vi "vectorAdd.vi"(2 "b":cluster{"xPos":dbl, "yPos":dbl, "Theta":dbl}={"xPos"=nan, "yPos"=nan, "Theta"=nan}, 3 "operation":enum16{"Subtract", "Add"}(ring), 4 "a":cluster{"xPos":dbl, "yPos":dbl, "Theta":dbl}={"xPos"=nan, "yPos"=nan, "Theta"=nan}) -> (1 "a +/- b":cluster{"xPos":dbl, "yPos":dbl, "Theta":dbl}={"xPos"=nan, "yPos"=nan, "Theta"=nan})   [LabVIEW 2016]
uses:
  <vilib>/Analysis/coordinate.llb/Angle Units.ctl
  <vilib>/Analysis/coordinate.llb/Angle Range (Degree).ctl
  <vilib>/Analysis/coordinate.llb/Wrap Angle (scalar).vi
  <vilib>/Analysis/NI_AAL_Angle.lvlib
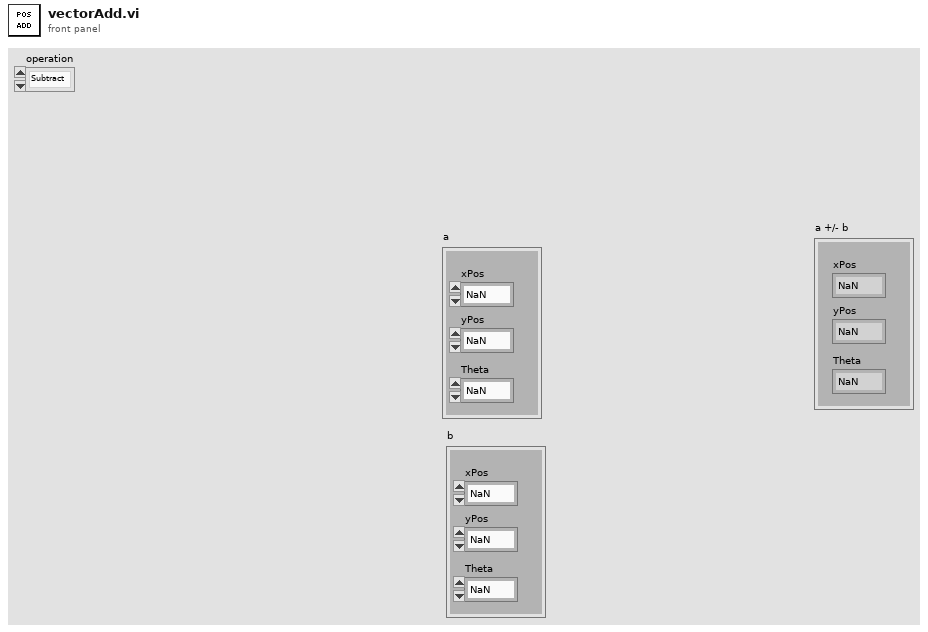
[diagram p1: front panel]
types:
  T1 = typedef "NI_AAL_Angle.lvlib/Angle Range (Degree).ctl" = u16
  T2 = typedef "NI_AAL_Angle.lvlib/Angle Units.ctl" = i32
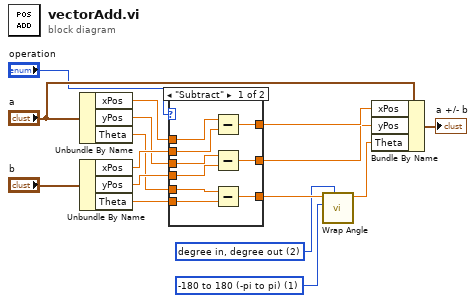
[diagram p0: block diagram]
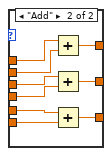
[diagram p2: hidden frame]
diagram:
  w2 = T1 1 items=["none", "-180 to 180 (-pi to pi)", "0 to 360 (0 to 2pi)"] ("angle range")
  w3 = T2 2 items=["radian in, radian out", "radian in, degree out", "degree in, degree out", "degree in, radian out"] ("angle units")
  n1 = Unbundle By Name("a") -> ("xPos"=w13:dbl, "yPos"=w10:dbl, "Theta"=w7:dbl)
  n2 = Unbundle By Name("b") -> ("xPos"=w12:dbl, "yPos"=w9:dbl, "Theta"=w6:dbl)
  n3 = case shown="\"Subtract\"" "operation" {
    tunnel: w13 -> [w25 w34]
    tunnel: w12 -> [w24 w33]
    tunnel: [w23 w32] -> w11
    tunnel: w10 -> [w22 w31]
    tunnel: w9 -> [w21 w30]
    tunnel: [w20 w29] -> w8
    tunnel: w7 -> [w19 w28]
    tunnel: w6 -> [w18 w27]
    tunnel: [w17 w26] -> w5
    frame "Subtract" {
      n4 = Subtract(x=w25, y=w24) -> (x-y=w23:dbl)
      n5 = Subtract(x=w22, y=w21) -> (x-y=w20:dbl)
      n6 = Subtract(x=w19, y=w18) -> (x-y=w17:dbl)
    }
    frame "Add" {
      n7 = Add(x=w34, y=w33) -> (x+y=w32:dbl)
      n8 = Add(x=w31, y=w30) -> (x+y=w29:dbl)
      n9 = Add(x=w28, y=w27) -> (x+y=w26:dbl)
    }
  }
  n10 = call-poly <vilib>:"Wrap Angle.vi"("angle units"=w3, "angle range"=w2, "angle in"=w5) -> ("angle out"=w4:dbl)  [unwired: 7 in, 1 out]
  n11 = Bundle By Name(cluster="a", "xPos"=w11, "yPos"=w8, "Theta"=w4) -> (→"a +/- b":cluster{"xPos":dbl, "yPos":dbl, "Theta":dbl})
